vi "ad get product info.vi"(7 "size":i32, 8 "error in (no error)":errorcluster, 9 "info":T1, 10 "id":i32, 11 "adh":i32) -> (0 "error out":errorcluster, 1 "info out":T1, 3 "function return":i32)   [LabVIEW 2021, in "libad4.lvlib"]
doc: "LIBAD4 function: ad_get_product_info (int32_t adh, int id, struct ad_product_info *info, int32_t size);\n\nReturns the serial number, firmware version, and the product name of the device associated with the passed device handle `adh`."
uses:
  <userlib>/libad4/libad4.lvlib
  <userlib>/libad4/controls/ad product info.ctl
  <userlib>/libad4/libad4.dll
types:
  T1 = typedef "libad4.lvlib/ad product info.ctl" = cluster{"serial":u32, "fw_version":u32, "model[0]":i8, "model[1]":i8, "model[2]":i8, "model[3]":i8, "model[4]":i8, "model[5]":i8, "model[6]":i8, "model[7]":i8, "model[8]":i8, "model[9]":i8, "model[10]":i8, "model[11]":i8, "model[12]":i8, "model[13]":i8, "model[14]":i8, "model[15]":i8, "model[16]":i8, "model[17]":i8, "model[18]":i8, "model[19]":i8, "model[20]":i8, "model[21]":i8, "model[22]":i8, "model[23]":i8, "model[24]":i8, "model[25]":i8, "model[26]":i8, "model[27]":i8, "model[28]":i8, "model[29]":i8, "model[30]":i8, "model[31]":i8, "res[0]":u8, "res[1]":u8, "res[2]":u8, "res[3]":u8, "res[4]":u8, "res[5]":u8, "res[6]":u8, "res[7]":u8, "res[8]":u8, "res[9]":u8, "res[10]":u8, "res[11]":u8, "res[12]":u8, "res[13]":u8, "res[14]":u8, "res[15]":u8, "res[16]":u8, "res[17]":u8, "res[18]":u8, "res[19]":u8, "res[20]":u8, "res[21]":u8, "res[22]":u8, "res[23]":u8, "res[24]":u8, "res[25]":u8, "res[26]":u8, "res[27]":u8, "res[28]":u8, "res[29]":u8, "res[30]":u8, "res[31]":u8, "res[32]":u8, "res[33]":u8, "res[34]":u8, "res[35]":u8, "res[36]":u8, "res[37]":u8, "res[38]":u8, "res[39]":u8, "res[40]":u8, "res[41]":u8, "res[42]":u8, "res[43]":u8, "res[44]":u8, "res[45]":u8, "res[46]":u8, "res[47]":u8, "res[48]":u8, "res[49]":u8, "res[50]":u8, "res[51]":u8, "res[52]":u8, "res[53]":u8, "res[54]":u8, "res[55]":u8, "res[56]":u8, "res[57]":u8, "res[58]":u8, "res[59]":u8, "res[60]":u8, "res[61]":u8, "res[62]":u8, "res[63]":u8, "res[64]":u8, "res[65]":u8, "res[66]":u8, "res[67]":u8, "res[68]":u8, "res[69]":u8, "res[70]":u8, "res[71]":u8, "res[72]":u8, "res[73]":u8, "res[74]":u8, "res[75]":u8, "res[76]":u8, "res[77]":u8, "res[78]":u8, "res[79]":u8, "res[80]":u8, "res[81]":u8, "res[82]":u8, "res[83]":u8, "res[84]":u8, "res[85]":u8, "res[86]":u8, "res[87]":u8, "res[88]":u8, "res[89]":u8, "res[90]":u8, "res[91]":u8, "res[92]":u8, "res[93]":u8, "res[94]":u8, "res[95]":u8, "res[96]":u8, "res[97]":u8, "res[98]":u8, "res[99]":u8, "res[100]":u8, "res[101]":u8, "res[102]":u8, "res[103]":u8, "res[104]":u8, "res[105]":u8, "res[106]":u8, "res[107]":u8, "res[108]":u8, "res[109]":u8, "res[110]":u8, "res[111]":u8, "res[112]":u8, "res[113]":u8, "res[114]":u8, "res[115]":u8, "res[116]":u8, "res[117]":u8, "res[118]":u8, "res[119]":u8, "res[120]":u8, "res[121]":u8, "res[122]":u8, "res[123]":u8, "res[124]":u8, "res[125]":u8, "res[126]":u8, "res[127]":u8, "res[128]":u8, "res[129]":u8, "res[130]":u8, "res[131]":u8, "res[132]":u8, "res[133]":u8, "res[134]":u8, "res[135]":u8, "res[136]":u8, "res[137]":u8, "res[138]":u8, "res[139]":u8, "res[140]":u8, "res[141]":u8, "res[142]":u8, "res[143]":u8, "res[144]":u8, "res[145]":u8, "res[146]":u8, "res[147]":u8, "res[148]":u8, "res[149]":u8, "res[150]":u8, "res[151]":u8, "res[152]":u8, "res[153]":u8, "res[154]":u8, "res[155]":u8, "res[156]":u8, "res[157]":u8, "res[158]":u8, "res[159]":u8, "res[160]":u8, "res[161]":u8, "res[162]":u8, "res[163]":u8, "res[164]":u8, "res[165]":u8, "res[166]":u8, "res[167]":u8, "res[168]":u8, "res[169]":u8, "res[170]":u8, "res[171]":u8, "res[172]":u8, "res[173]":u8, "res[174]":u8, "res[175]":u8, "res[176]":u8, "res[177]":u8, "res[178]":u8, "res[179]":u8, "res[180]":u8, "res[181]":u8, "res[182]":u8, "res[183]":u8, "res[184]":u8, "res[185]":u8, "res[186]":u8, "res[187]":u8, "res[188]":u8, "res[189]":u8, "res[190]":u8, "res[191]":u8, "res[192]":u8, "res[193]":u8, "res[194]":u8, "res[195]":u8, "res[196]":u8, "res[197]":u8, "res[198]":u8, "res[199]":u8, "res[200]":u8, "res[201]":u8, "res[202]":u8, "res[203]":u8, "res[204]":u8, "res[205]":u8, "res[206]":u8, "res[207]":u8, "res[208]":u8, "res[209]":u8, "res[210]":u8, "res[211]":u8, "res[212]":u8, "res[213]":u8, "res[214]":u8, "res[215]":u8, "res[216]":u8, "res[217]":u8, "res[218]":u8, "res[219]":u8, "res[220]":u8, "res[221]":u8, "res[222]":u8, "res[223]":u8, "res[224]":u8, "res[225]":u8, "res[226]":u8, "res[227]":u8, "res[228]":u8, "res[229]":u8, "res[230]":u8, "res[231]":u8, "res[232]":u8, "res[233]":u8, "res[234]":u8, "res[235]":u8, "res[236]":u8, "res[237]":u8, "res[238]":u8, "res[239]":u8, "res[240]":u8, "res[241]":u8, "res[242]":u8, "res[243]":u8, "res[244]":u8, "res[245]":u8, "res[246]":u8, "res[247]":u8, "res[248]":u8, "res[249]":u8, "res[250]":u8, "res[251]":u8, "res[252]":u8, "res[253]":u8, "res[254]":u8, "res[255]":u8}
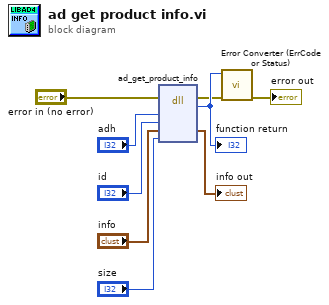
[diagram p0: block diagram]
diagram:
  n1 = dll-call lib="C:/Program Files/National Instruments/LabVIEW 2021/user.lib/libad4/libad4.*" fn="ad_get_product_info"(error in="error in (no error)", "adh"="adh", "id"="id", "info"="info", "size"="size") -> (error out=w2:errorcluster, w9:i32, "info"=→"info out":T1)  [unwired: 5 in, 1 out]
  "function return" <- w9
  n2 = call <userlib>:"Error Converter (ErrCode or Status).vi"("error in (no error)"=w2, "error code"=w9) -> ("error out"=→"error out":errorcluster)  [unwired: 9 in]
